vi "Controller error.vi"() -> ()   [LabVIEW 2010]
panel:
  in  "Cluster":T1 {"Module erro mask" format="%.0x"}
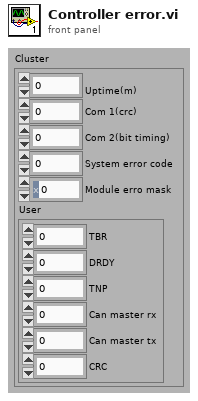
[diagram p1: front panel]
types:
  T1 = cluster{"Uptime(m)":u16, "Com 1(crc)":u8, "Com 2(bit timing)":u8, "System error code":u8, "Module erro mask":u8, "User":cluster{"TBR":u16, "DRDY":u16, "TNP":u16, "Can master rx":u16, "Can master tx":u16, "CRC":u16}}
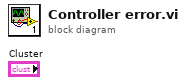
[diagram p0: block diagram]
diagram:
